vi "Write Glue Step Enum.vi"(8 "error in (no error)":errorcluster, 10 "Glue Step Enum":T1, 11 "Iterative Dispense in":refnum<class "Iterative Dispense.lvclass">) -> (0 "error out":errorcluster, 3 "Iterative Dispense out":refnum<class "Iterative Dispense.lvclass">)   [LabVIEW 2021, in "Iterative Dispense.lvclass"]
uses:
  Iterative Dispense.lvclass
  Glue Step Enum.ctl
  Iterative Dispense.lvclass/Iterative Dispense.ctl
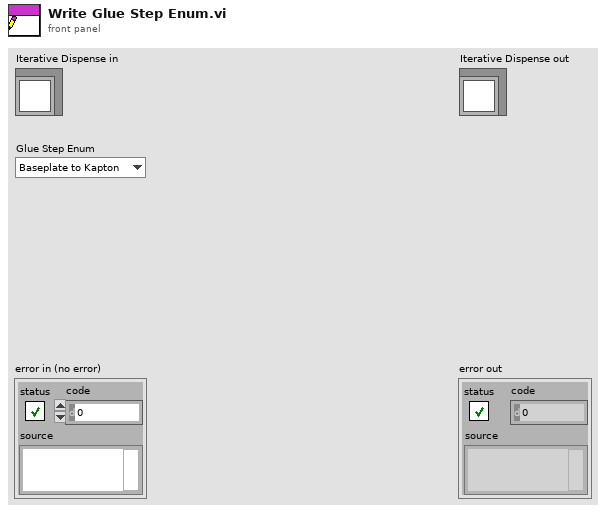
[diagram p1: front panel]
types:
  T1 = typedef "Iterative Dispense.lvclass/Glue Step Enum.ctl" = enum16{"Baseplate to Kapton", "Kapton to Sensor"}
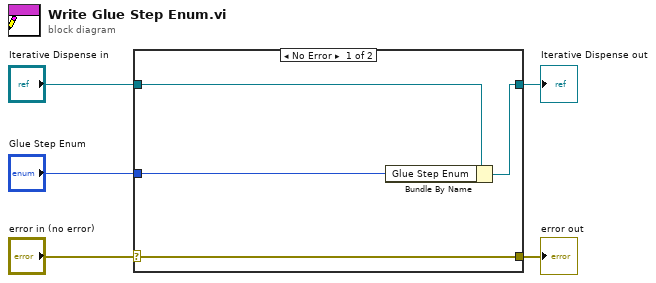
[diagram p0: block diagram]
diagram:
  n1 = case shown="No Error" "error in (no error)" {
    selector: "error in (no error)" -> [w9 w10]
    tunnel: [w9 w10] -> w4
    tunnel: [w7 w11] -> w2
    tunnel: "Iterative Dispense in" -> [w8 w11]
    tunnel: "Glue Step Enum" -> [w6 _]
    frame No Error {
      n2 = Bundle By Name(cluster=w8, "Glue Step Enum"=w6) -> (w7:refnum<class "Iterative Dispense.lvclass">)
    }
    frame Error {
    }
  }
  "error out" <- w4
  "Iterative Dispense out" <- w2
